vi "Initialize Subscription Policy.vi"(9 "Last Publish Time":timestamp, 10 "Last Topic Value":variant, 11 "Subscription Policy":T1) -> (0 "Error Out (Do Not Subscribe?)":errorcluster)   [LabVIEW 2017, in "IMediator.lvlib" / "ISubscriptionPolicy.lvclass"]
doc: "This method decides whether or not to send or otherwise handle the new data value. The policy is set and maintained by the subscriber. The Topic Actor knows no policy details, it just passes the new value in. If there is a failure inside this method, the Topic Actor must assume the listener is no longer valid (dead/unrecoverable) and should delete it from the Subscriber list.\n\n<License>\nCopyright © 2017 Composed Systems, LLC | All rights reserved\nwww.composed.io\n\nAuthor: Ethan Stern <ethan.stern@composed.io>\n\nThis software is provided \"AS IS\" WITHOUT WARRANTIES, either express or implied, AND IS FOR EDUCATIONAL PURPOSES ONLY.\n</License>"
uses:
  ISubscriptionPolicy.lvclass
  ISubscriptionPolicy Reference.ctl
  ISubscriptionPolicy.lvclass/ISubscriptionPolicy.ctl
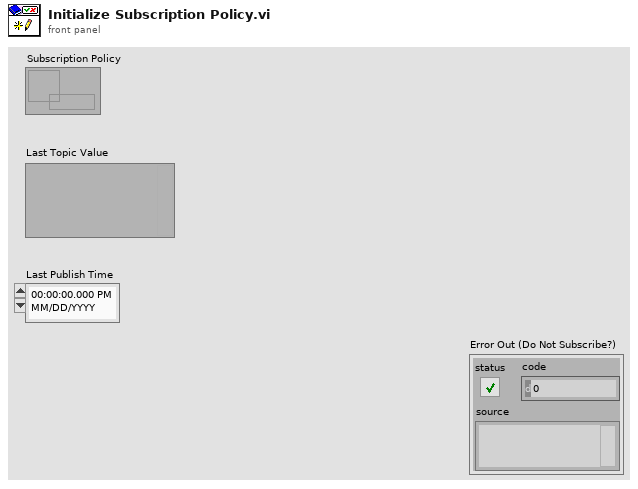
[diagram p1: front panel]
types:
  T1 = typedef "IMediator.lvlib/ISubscriptionPolicy.lvclass/ISubscriptionPolicy Reference.ctl" = refnum<data-value>
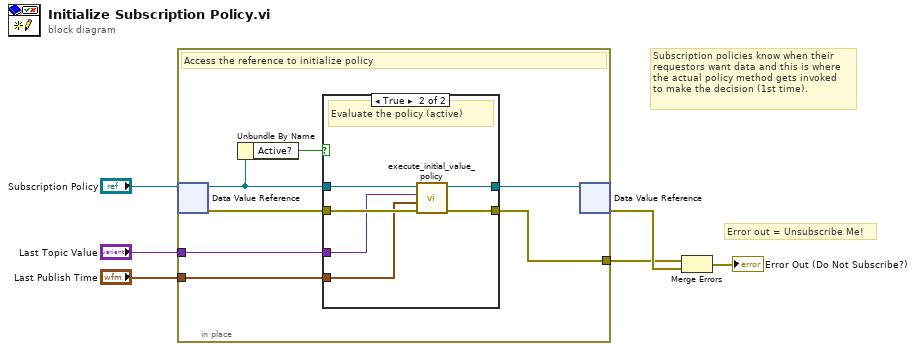
[diagram p0: block diagram]
diagram:
  # "Error out = Unsubscribe Me!"
  # "Subscription policies know when their\nrequestors want data and this is where\nthe actual policy method gets invoked\nto make the decision (1st time)."
  n1 = in-place {
    in-place-border: "Last Topic Value" -> [w11]
    in-place-border: "Last Publish Time" -> [w10]
    in-place-border: [w9] -> w2
    # "Access the reference to initialize policy"
    n2 = in-place-dvr #1("Subscription Policy") -> (w8:refnum<class "ISubscriptionPolicy.lvclass">, w12:errorcluster)
    n3 = Unbundle By Name(w8) -> ("Active?"=w7:bool)
    n4 = case shown="True" w7 {
      tunnel: w8 -> [w15 w21]
      tunnel: [w15 w20] -> w13
      tunnel: w12 -> [w14 w19]
      tunnel: w11 -> [_ w18]
      tunnel: w10 -> [_ w17]
      tunnel: [w14 w16] -> w9
      frame False {
        # "Skip evaluation (not active)"
      }
      frame True {
        # "Evaluate the policy (active)"
        n5 = call-dynamic "execute_initial_value_policy.vi"("error in (no error)"=w19, "Last Publish Time"=w17, "Last Topic Value"=w18, "ISubscriptionPolicy In"=w21) -> ("error out"=w16:errorcluster, "ISubscriptionPolicy Out"=w20:refnum<class "ISubscriptionPolicy.lvclass">)  [unwired: 6 in]
      }
    }
    n6 = in-place-dvr #1(w13) -> (w3:errorcluster)  [unwired: 1 out]
  }
  n7 = Merge Errors(w2, w3) -> (→"Error Out (Do Not Subscribe?)":errorcluster)
